vi "all of.vi"(11 "Device ID":T1(ring)) -> ()   [LabVIEW 2010]
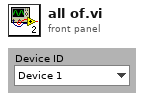
[diagram p1: front panel]
types:
  T1 = enum16{"Device 1", "Device 2", "Device 3", "Device 4", "Device 5", "Device 6", "Device 7", "Device 8"}
  T2 = enum8{"Power 1", "Power 2", "Power 3", "Power 4", "Power 5", "Power 6", "Power 7", "Power 8"}
  T3 = enum8{"Output 1 (O1)", "Output 2 (O2)", "Output 3 (O3)", "Output 4 (O4)", "Output 5 (O5)", "Output 6 (O6)", "Output 7 (O7)", "Output 8 (O8)"}[]
  T4 = enum8{"Robo Interface", "Extension 1", "Extension 2", "Extension 3"}[]
  T5 = enum8{"Power 1", "Power 2", "Power 3", "Power 4", "Power 5", "Power 6", "Power 7", "Power 8"}[]
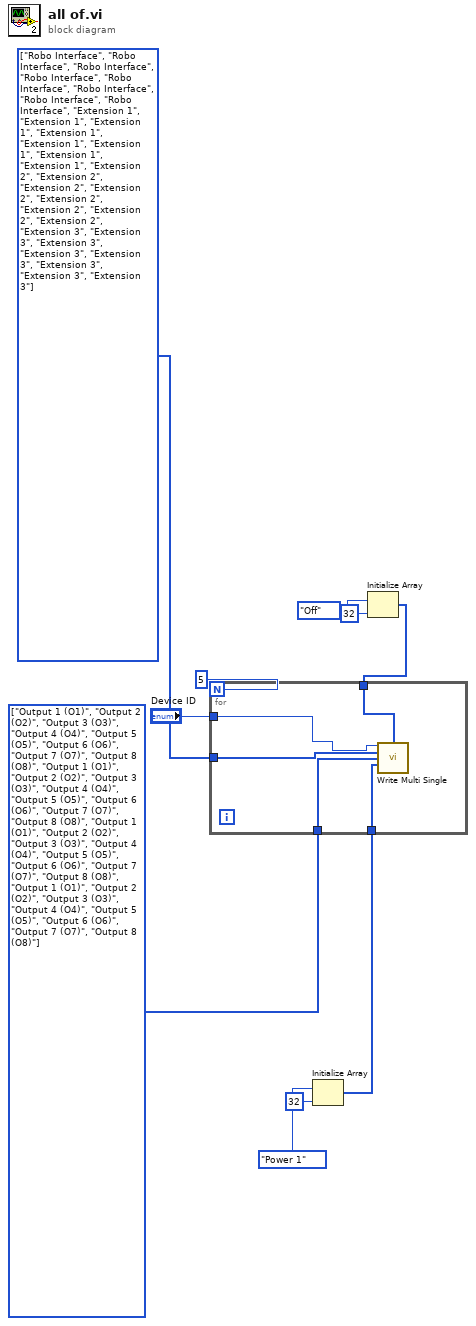
[diagram p0: block diagram]
diagram:
  w7 = T3 [enum."Output 1 (O1)", enum."Output 2 (O2)", enum."Output 3 (O3)", enum."Output 4 (O4)", enum."Output 5 (O5)", enum."Output 6 (O6)", enum."Output 7 (O7)", enum."Output 8 (O8)", enum."Output 1 (O1)", enum."Output 2 (O2)", enum."Output 3 (O3)", enum."Output 4 (O4)", enum."Output 5 (O5)", enum."Output 6 (O6)", enum."Output 7 (O7)", enum."Output 8 (O8)", enum."Output 1 (O1)", enum."Output 2 (O2)", enum."Output 3 (O3)", enum."Output 4 (O4)", enum."Output 5 (O5)", enum."Output 6 (O6)", enum."Output 7 (O7)", enum."Output 8 (O8)", enum."Output 1 (O1)", enum."Output 2 (O2)", enum."Output 3 (O3)", enum."Output 4 (O4)", enum."Output 5 (O5)", enum."Output 6 (O6)", enum."Output 7 (O7)", enum."Output 8 (O8)"] items=["Output 1 (O1)", "Output 2 (O2)", "Output 3 (O3)", "Output 4 (O4)", "Output 5 (O5)", "Output 6 (O6)", "Output 7 (O7)", "Output 8 (O8)"] ("Single_Output")
  w8 = T4 [enum."Robo Interface", enum."Robo Interface", enum."Robo Interface", enum."Robo Interface", enum."Robo Interface", enum."Robo Interface", enum."Robo Interface", enum."Robo Interface", enum."Extension 1", enum."Extension 1", enum."Extension 1", enum."Extension 1", enum."Extension 1", enum."Extension 1", enum."Extension 1", enum."Extension 1", enum."Extension 2", enum."Extension 2", enum."Extension 2", enum."Extension 2", enum."Extension 2", enum."Extension 2", enum."Extension 2", enum."Extension 2", enum."Extension 3", enum."Extension 3", enum."Extension 3", enum."Extension 3", enum."Extension 3", enum."Extension 3", enum."Extension 3", enum."Extension 3"] items=["Robo Interface", "Extension 1", "Extension 2", "Extension 3"] ("Module")
  n1 = Initialize Array(T2."Power 1" ("Output_PWM"), 32 ("Dimension")) -> (w1:T5)
  n2 = Initialize Array(enum8{"Off", "On"}."Off" ("Output_Action"), 32 ("Dimension")) -> (w4:enum8{"Off", "On"}[])
  n3 = for {
    N: 5 -> [_]
    tunnel: "Device ID" -> [w15]
    tunnel: w8 -> [w14]
    tunnel: w7 -> [w13]
    tunnel: w4 -> [w12]
    tunnel: w1 -> [w11]
    n4 = call "Write Multi Single.vi"("Device ID"=w15, "Output_Action"=w12, "Module"=w14, "Single_Output"=w13, "Output_PWM"=w11) -> ()  [unwired: 1 in, 10 out]
  }
